vi "FIFOStopDAQ.vi"() -> (0 "error out":errorcluster)   [LabVIEW 2009]
uses:
  hhlib.dll
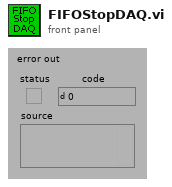
[diagram p1: front panel]
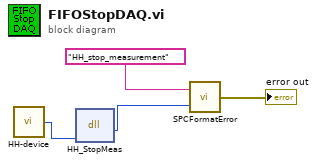
[diagram p0: block diagram]
diagram:
  n1 = call "HH-device.vi"() -> ("Device (output)"=w1:i32)  [unwired: 2 in]
  n2 = dll-call lib="C:/Programme/Anwendungen/DAQLinescan_HH/hhlib.dll" fn="HH_StopMeas"("devidx"=w1) -> (w2:i32)  [unwired: 4 in, 2 out]
  n3 = call "SPCFormatError.vi"("Error Code"=w2, "Source"="HH_stop_measurement") -> ("error out"=→"error out":errorcluster)
